vi "find_spectral_peaks.vi"(4 "Min ampl":dbl, 6 "Freq filter":dbl=-1.0, 7 "Fs":dbl=2.0, 10 "Complex Spectrum":cdb[](array[numeric]), 11 "Freq res":dbl) -> (3 "Peaks":dbl[][](array[numeric]))   [LabVIEW 2012]
uses:
  <vilib>/Analysis/coordinate.llb/Wrap Angle (array).vi
  <vilib>/Analysis/NI_AAL_Angle.lvlib
panel:
  # "Return only components that alias to this frequency.  If negative, return all components."
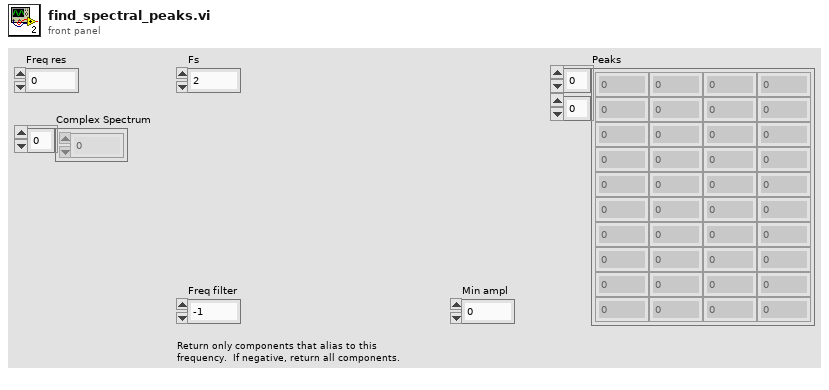
[diagram p1: front panel]
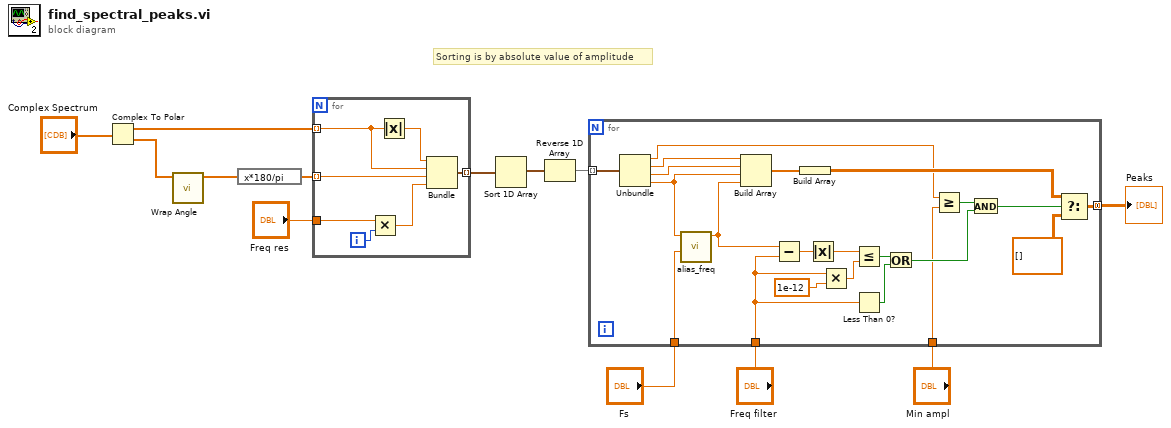
[diagram p0: block diagram]
diagram:
  # "Sorting is by absolute value of amplitude"
  n1 = Complex To Polar(r * e^(i*theta)="Complex Spectrum") -> (r=w4:dbl[], theta=w2:dbl[])
  n2 = call-poly <vilib>:"Wrap Angle.vi"("Angle In"=w2) -> ("Angle Out"=w1:dbl[])  [unwired: 9 in, 1 out]
  n3 = expression code="x*180/pi"(w1) -> (w5:dbl[])
  n4 = for {
    tunnel: w4 -> [w14] mode=indexing
    tunnel: "Freq res" -> [w20]
    tunnel: [w17] -> w12 mode=indexing
    tunnel: w5 -> [w16] mode=indexing
    i -> [w19]
    n5 = Multiply(x=w20, y=w19) -> (x*y=w18:dbl)
    n6 = Absolute Value(x=w14) -> (abs(x)=w15:dbl)
    n7 = Bundle(w15, w14, "Numeric"=w16, w18) -> (w17:cluster{dbl, dbl, "Numeric":dbl, dbl})  [unwired: 1 in]
  }
  n8 = Sort 1D Array(array=w12) -> (sorted array=w11:cluster{dbl, dbl, "Numeric":dbl, dbl}[])
  n9 = Reverse 1D Array(array=w11) -> (reversed array=w10:cluster{dbl, dbl, "Numeric":dbl, dbl}[])
  n10 = for {
    tunnel: w10 -> [w28] mode=indexing
    tunnel: "Fs" -> [w42]
    tunnel: [w34] -> w8 mode=concatenating
    tunnel: "Freq filter" -> [w22]
    tunnel: "Min ampl" -> [w30]
    n11 = Unbundle(w28) -> (w24:dbl, w25:dbl, "Numeric"=w26:dbl, w27:dbl)
    n12 = call "alias_freq.vi"("Fs"=w42, "F"=w27) -> ("F aliased"=w40:dbl)  [unwired: 9 in]
    n13 = Build Array(w25, w26, w27, w40) -> (w37:dbl[])
    n14 = Subtract(x=w40, y=w22) -> (x-y=w39:dbl)
    n15 = Build Array(w37) -> (w36:dbl[][])
    n16 = Absolute Value(x=w39) -> (abs(x)=w33:dbl)
    n17 = Multiply(x=w22, y=1e-12) -> (x*y=w23:dbl)
    n18 = Less Or Equal?(x=w33, y=w23) -> (x <= y?=w38:bool)
    n19 = Less Than 0?(x=w22) -> (x < 0?=w41:bool)
    n20 = Or(x=w38, y=w41) -> (x .or. y?=w32:bool)
    n21 = Greater Or Equal?(x=w24, y=w30) -> (x >= y?=w29:bool)
    n22 = And(x=w29, y=w32) -> (x .and. y?=w31:bool)
    n23 = Select(t=w36, s=w31, f=dbl[][] []) -> (s? t:f=w34:dbl[][])
  }
  "Peaks" <- w8
